vi "Timed relay switch and delay.vi"() -> ()   [LabVIEW 2017]
uses:
  <vilib>/Platform/TimedLoop/XDataNode/timing_clust.ctl
  <vilib>/Platform/TimedLoop/XDataNode/nitl_modes.ctl
  <vilib>/Platform/TimedLoop/XDataNode/wakeup.ctl
  <vilib>/DAQmx/write.llb/DAQmx Write (Digital Bool 1Line 1Point).vi
  <vilib>/DAQmx/create/channels.llb/DAQmx Create Channel (DO-Digital Output).vi
  <vilib>/DAQmx/miscellaneous.llb/DAQmx Fill In Error Info.vi
  <vilib>/Platform/TimedLoop/XDataNode/XDataNode.xnode
  <vilib>/Platform/TimedLoop/XDataNode/XDNodeRunTimeDep.lvlib
panel:
  in  "Off Time":dbl
  in  "stop":bool
  in  "On Time":i64=1000
  out "counter":i8
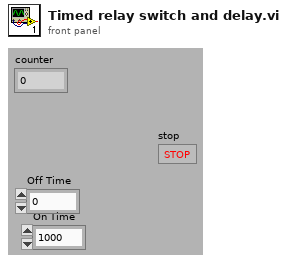
[diagram p1: front panel]
types:
  T1 = typedef "XDNodeRunTimeDep.lvlib/timing_clust.ctl" = cluster{"Expected End [f-1]":u64, "Actual End [f-1]":u64, "Finished Late? [f-1]":bool, "Expected End [i-1]":u64, "Actual End [i-1]":u64, "Finished Late? [i-1]":bool, "Expected Start [i]":u64, "Actual Start [i]":u64, "Expected Start [f]":u64, "Actual Start [f]":u64, "Source Name":string, "Structure Name":string, "Period":i64, "Deadline":i64, "Offset":i64, "Start":i64, "Priority":i32, "Timeout":i32, "Mode":T2, "Wakeup Reason":T3, "Error":errorcluster, "Source Type":string, "Secondary Source Type":string, "Global End Time":u64, "Global Start Time":u64, "Frame Duration":u64, "Iteration Duration":u64, "Assigned CPU":i32, "I/O Scan Engine Mode":u32}
  T2 = typedef "XDNodeRunTimeDep.lvlib/nitl_modes.ctl" = enum32{"No Change", "Process missed periods, maintain original phase", "Discard missed periods, maintain original phase", "Process missed periods, ignore original phase", "Discard missed periods, ignore original phase"}
  T3 = typedef "XDNodeRunTimeDep.lvlib/wakeup.ctl" = enum32{"Normal", "Aborted", "Asynchronous wakeup", "Timing source error", "Timed loop error", "Timeout"}
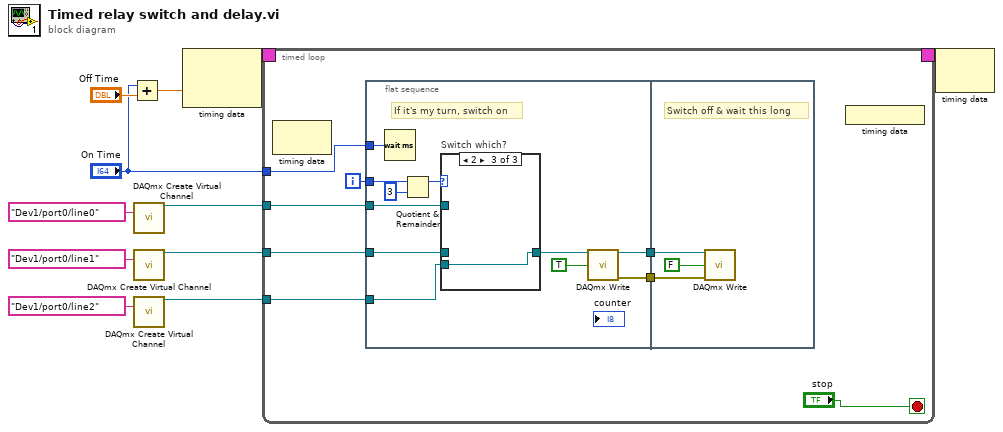
[diagram p0: block diagram]
diagram:
  n1 = Add(x="On Time", y="Off Time") -> (x+y=w2:dbl)
  n2 = call-poly <vilib>:"DAQmx Create Virtual Channel.vi"("lines"=tag "Dev1/port0/line0") -> ("task out"=w8:refnum<k21>)  [unwired: 5 in, 9 out]
  n3 = call-poly <vilib>:"DAQmx Create Virtual Channel.vi"("lines"=tag "Dev1/port0/line1") -> ("task out"=w7:refnum<k21>)  [unwired: 5 in, 9 out]
  n4 = call-poly <vilib>:"DAQmx Create Virtual Channel.vi"("lines"=tag "Dev1/port0/line2") -> ("task out"=w6:refnum<k21>)  [unwired: 5 in, 9 out]
  n5 = node-c288(w2) -> (w5:T1)  [unwired: 1 out]
  n6 = timed-loop {
    timing: w5 -> [_]
    timing-out: [_] -> w4
    tunnel: w6 -> [w18]
    tunnel: w7 -> [w17]
    tunnel: w8 -> [w15]
    tunnel: "On Time" -> [w16]
    i -> [w13]
    stop <- "stop" stop-if-true
    n7 = node-c288() -> ()  [unwired: 2 out]
    n8 = flat-sequence {
      tunnel: w18 -> [w22]
      tunnel: w17 -> [w21]
      tunnel: w15 -> [w27]
      tunnel: w16 -> [w30]
      tunnel: [w28] -> w14
      tunnel: w13 -> [w23]
      tunnel: [w20] -> w12
      tunnel: w14 -> [w35]
      tunnel: w12 -> [w34]
      frame #0 {
        # "If it's my turn, switch on"
        n9 = Wait (ms)(milliseconds to wait=w30) -> ()  [unwired: 1 out]
        n10 = Quotient & Remainder(x=w23, y=3) -> (x-y*floor(x/y)=w24:i32)  [unwired: 1 out]
        n11 = case "Switch which?" shown="2" w24 {
          tunnel: w27 -> [w31 _ _]
          tunnel: [w31 w32 w33] -> w26
          tunnel: w22 -> [_ _ w33]
          tunnel: w21 -> [_ w32 _]
          frame 0, Default {
          }
          frame 1 {
          }
          frame 2 {
          }
        }
        n12 = call-poly <vilib>:"DAQmx Write.vi"("task/channels in"=w26, "data"=TRUE) -> ("task out"=w28:refnum<k21>, "error out"=w20:errorcluster)  [unwired: 2 in, 10 out]
      }
      frame #1 {
        # "Switch off & wait this long"
        n13 = call-poly <vilib>:"DAQmx Write.vi"("task/channels in"=w35, "data"=FALSE, "error in"=w34) -> ()  [unwired: 1 in, 12 out]
      }
    }
    n14 = node-c288() -> ()  [unwired: 1 out]
  }
  n15 = node-c288(w4) -> ()  [unwired: 1 out]
